vi "GetEvtReports.vi"(8 "error in (no error)":errorcluster, 11 "RngEventPlugin in":refnum<class "C37EvtPlugin.lvclass">) -> (0 "error out":errorcluster, 3 "C37EventPlugin out":refnum<class "C37EvtPlugin.lvclass">)   [LabVIEW 2017, in "EventPlugins.lvlib" / "C37EvtPlugin.lvclass"]
uses:
  C37EvtPlugin.lvclass
  C:/dev/Work/PARTF/Modules/EventPlugins/EventPluginBaseClass/EventPluginBaseClass.lvclass
  EventPluginBaseClass/EventPluginBaseClass.lvclass/EventPluginBaseClass.ctl
  EventPluginBaseClass/TypeDefs/clEvtReport.ctl
  EventPluginBaseClass/Accessors/Read BusNumber.vi
  EventPluginBaseClass/Accessors/Read EvtConfig.vi
  EventPluginBaseClass/Accessors/Read TimeArray.vi
  EventPluginBaseClass/Accessors/Read EvtParams.vi
  EventPluginBaseClass/EventPluginBaseClass.lvclass
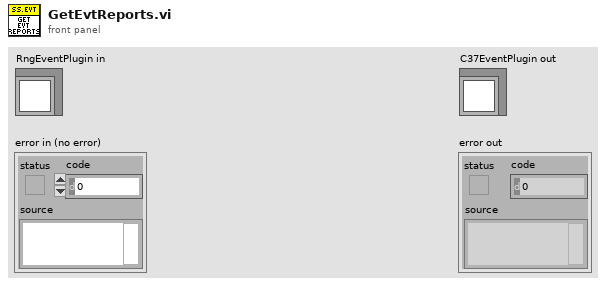
[diagram p1: front panel]
types:
  T1 = typedef "EventPlugins.lvlib/EventPluginBaseClass.lvclass/clEvtReport.ctl" = cluster{"Timestamp":dbl, "Synx":cdb[], "Freq":dbl, "ROCOF":dbl, "ID":i16}
  T2 = typedef "EventPlugins.lvlib/EventPluginBaseClass.lvclass/clEvtConfig.ctl" = cluster{"T0(UTC)":dbl, "F0":dbl, "Fs":i32, "FSamp":u32, "bPosSeq":bool}
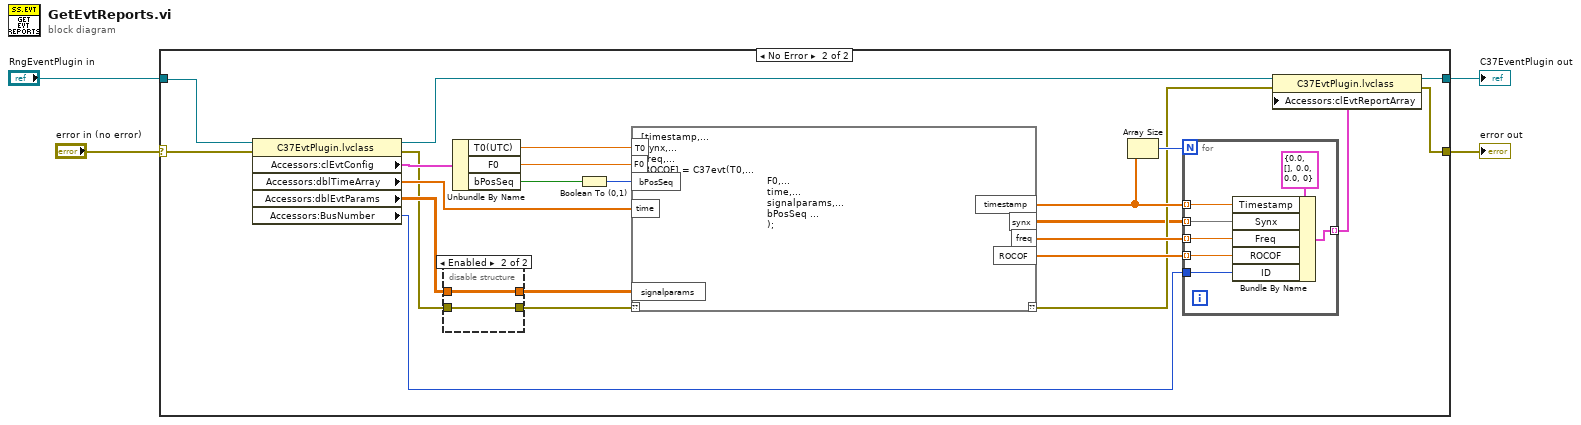
[diagram p0: block diagram]
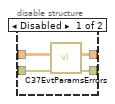
[diagram p3: hidden frame]
diagram:
  n1 = case shown="No Error" "error in (no error)" {
    selector: "error in (no error)" -> [w6 w24]
    tunnel: [w5 w27] -> w4
    tunnel: "RngEventPlugin in" -> [w5 w25]
    tunnel: [w6 w26] -> w3
    frame Error {
    }
    frame No Error {
      n2 = property class="C37EvtPlugin.lvclass"(reference=w25, error in=w24) -> (reference out=w20:refnum<class "C37EvtPlugin.lvclass">, error out=w10:errorcluster, "Accessors:clEvtConfig"=w23:T2, "Accessors:dblTimeArray"=w14:dbl[], "Accessors:dblEvtParams"=w11:dbl[][], "Accessors:BusNumber"=w8:u8)
      n3 = disable-structure shown="Enabled" {
        disable-tunnel: [w33 w34] -> w13
        disable-tunnel: [w32 w35] -> w12
        disable-tunnel: w11 -> [w31 w35]
        disable-tunnel: w10 -> [w30 w34]
        frame Disabled {
          n4 = call "C37EvtParamsErrors.vi"("error in (no error)"=w30, "dblSignalParams in"=w31) -> ("error out"=w33:errorcluster, "dblSignalParams out"=w32:dbl[][])  [unwired: 8 in]
        }
        frame Enabled {
        }
      }
      n5 = Unbundle By Name(w23) -> ("T0(UTC)"=w22:dbl, "F0"=w21:dbl, "bPosSeq"=w9:bool)
      n6 = Boolean To (0,1)(Boolean=w9) -> (0, 1=w7:i16)
      n7 = script code="[timestamp,...\n synx,...\n freq,...\n ROCOF] = C37evt(T0,...\n                                          F0,...\n                                          time,...\n                                          signalparams,...\n                                          bPosSeq ...\n                                          );"("??"=w13, "T0"=w22, "F0"=w21, "bPosSeq"=w7, "time"=w14, "signalparams"=w12) -> ("??"=w17:errorcluster, "timestamp"=w19:dbl[], "synx"=w16:cdb[][], "freq"=w29:dbl[], "ROCOF"=w28:dbl[])
      n8 = Array Size(array=w19) -> (size(s)=w18:i32)
      n9 = for {
        N: w18 -> [_]
        tunnel: w19 -> [w42] mode=indexing
        tunnel: w29 -> [w41] mode=indexing
        tunnel: w28 -> [w40] mode=indexing
        tunnel: [w38] -> w15 mode=indexing
        tunnel: w16 -> [w37] mode=indexing
        tunnel: w8 -> [w36]
        n10 = Bundle By Name(cluster=T1 {"Timestamp"=0.0, "Synx"=[], "Freq"=0.0, "ROCOF"=0.0, "ID"=0} ("clReport"), "Timestamp"=w42, "Synx"=w37, "Freq"=w41, "ROCOF"=w40, "ID"=w36) -> (w38:T1)
      }
      n11 = property class="C37EvtPlugin.lvclass"(reference=w20, error in=w17, "Accessors:clEvtReportArray"=w15) -> (reference out=w27:refnum<class "C37EvtPlugin.lvclass">, error out=w26:errorcluster)
    }
  }
  "error out" <- w3
  "C37EventPlugin out" <- w4
